vi "Revision Query Core.vi"(8 "error in (no error)":errorcluster, 11 "IVI_Fgen in":refnum<class "IVI_Fgen.lvclass">) -> (0 "error out":errorcluster, 1 "Firmware Revision":string, 2 "Driver Revision":string, 3 "IVI_Fgen out":refnum<class "IVI_Fgen.lvclass">)   [LabVIEW 2016, in "IVI_Fgen.lvlib" / "IVI_Fgen.lvclass"]
uses:
  IVI_Fgen.lvclass
  IVI_Fgen.lvclass/IVI_Fgen.ctl
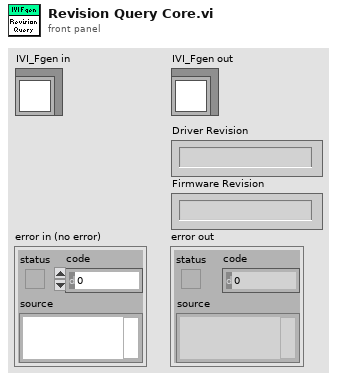
[diagram p1: front panel]
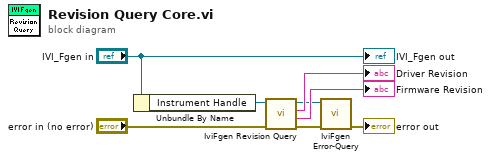
[diagram p0: block diagram]
diagram:
  n1 = Unbundle By Name("IVI_Fgen in") -> ("Instrument Handle"=w7:refnum<k15>)
  n2 = call <vilib>:"IviFgen Revision Query.vi"("error in (no error)"="error in (no error)", "instrument handle"=w7) -> ("error out"=w2:errorcluster, "firmware revision"=→"Firmware Revision":string, "instrument driver revision"=→"Driver Revision":string, "instrument handle out"=w3:refnum<k15>)  [unwired: 6 in]
  n3 = call <vilib>:"IviFgen Error-Query.vi"("error in (no error)"=w2, "instrument handle"=w3) -> ("error out"=→"error out":errorcluster)  [unwired: 6 in, 3 out]
  "IVI_Fgen out" <- "IVI_Fgen in"
